vi "obstacle expansion.vi"() -> ()   [LabVIEW 2010]
uses:
  4-High Neurons/4.1.2-Act Neuron TD.ctl
  3.0 Flow Control/3.0 List of Loops.ctl
  3.0-Global.vi
panel:
  out "Input Act Neurons":T1
  out "Heartbeat":bool
  out "Dont Run!":bool
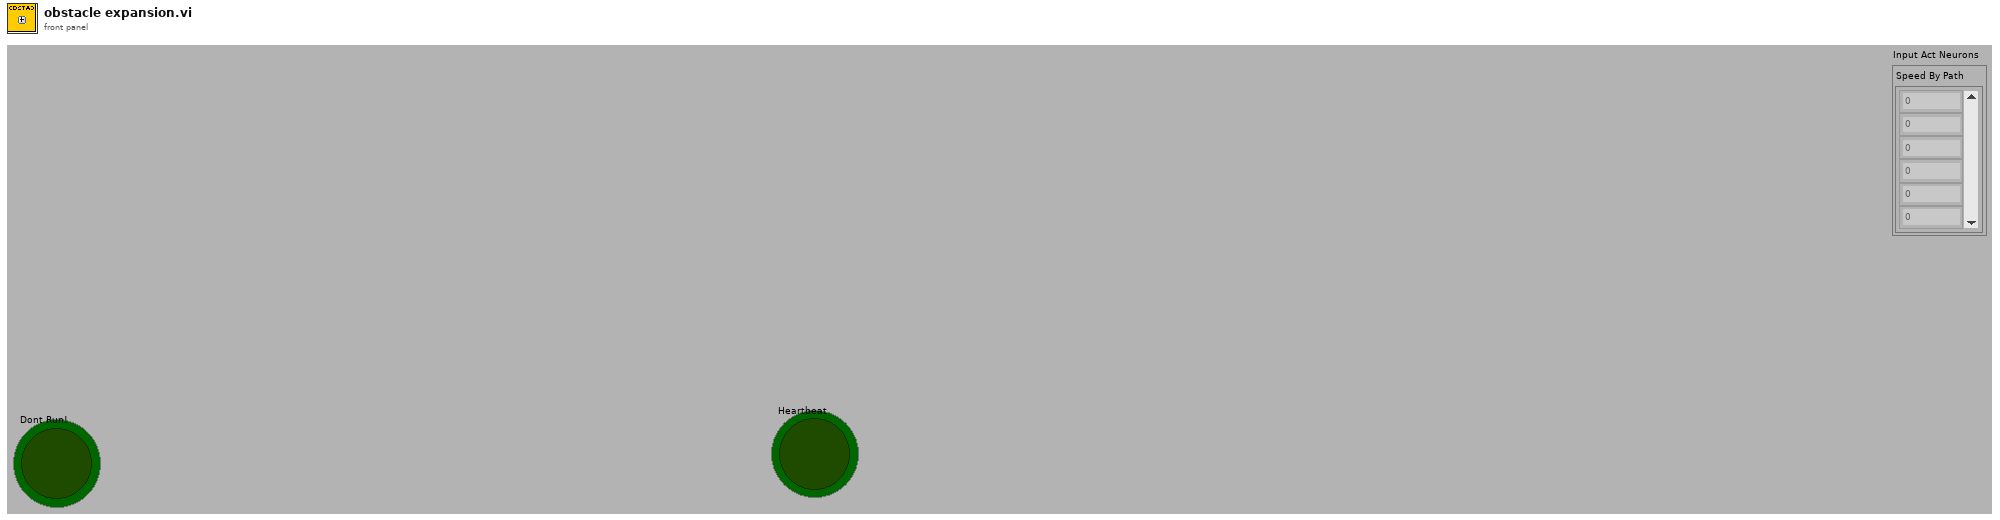
[diagram p1: front panel]
types:
  T1 = typedef "4.1.2-Act Neuron TD.ctl" = cluster{"Speed By Path":sgl[]}
  T2 = enum16{"Set Joystick", "Read Joystick", "Set Forebrain", "Read Forebrain", "Set Limbic", "Read Limbic", "Set Cerebellum", "Read Cerebellum", "Set Arbitrated", "Read Arbitrated", "Set LIDAR", "Read LIDAR"}
  T3 = typedef "3.0 List of Loops.ctl" = enum16{"3.0 State Update", "3.0 GUI", "3.1 Act", "3.1 4.7.1 Act UDP", "3.1 Joystick", "3.2 Where", "3.2 4.7.2 Where UDP", "3.3 What", "3.3 4.7.3 What UDP", "3.4 How", "3.4 4.7.4 How UDP", "3.5 Limbic", "3.8 TCP", "3.6 Cerebellum", "3.8 TCP Act"}
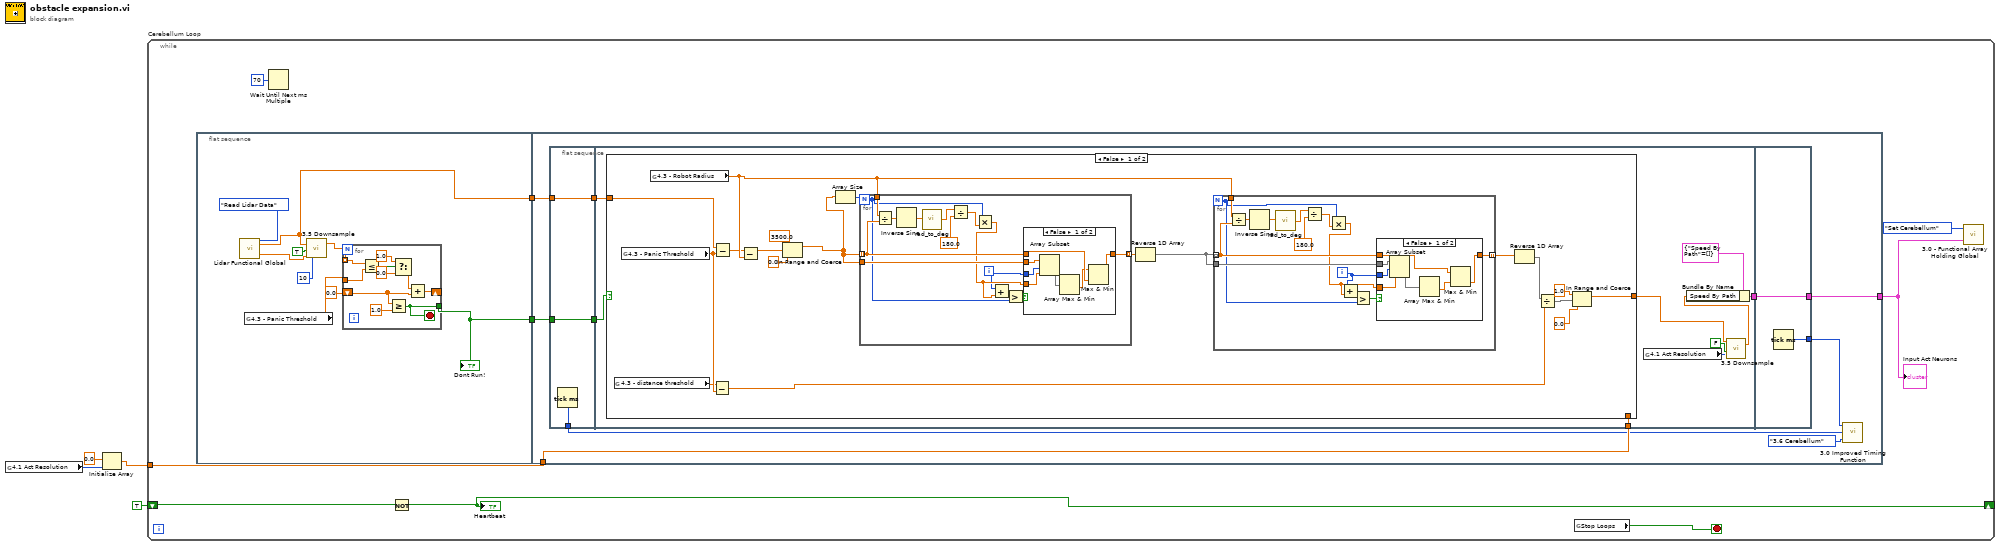
[diagram p0: block diagram]
diagram:
  n1 = global read "3.0-Global.vi" "4.1 Act Resolution"() -> (w2:u32)
  n2 = Initialize Array(0.0 ("element"), w2) -> (w1:dbl[])
  n3 = while "Cerebellum Loop" {
    shift-right: [w10] -> _
    shift-left: TRUE -> [w9]
    tunnel: w1 -> [w8]
    stop <- w11 stop-if-true
    n4 = flat-sequence {
      tunnel: [w15] -> w13
      tunnel: [w16] -> w12
      tunnel: w13 -> [w41]
      tunnel: w12 -> [w42]
      tunnel: w8 -> [w40]
      tunnel: [w39] -> w6
      frame #0 {
        n5 = call "Lidar Functional Global.vi"("Lidar Action"=enum16{"Set Lidar Data", "Read Lidar Data"}."Read Lidar Data") -> ("Lidar Angle Data Out (Degrees)"=w14:sgl[], "Lidar Magnitude Data Out (mm)"=w15:sgl[])  [unwired: 2 in]
        n6 = global read "3.0-Global.vi" "4.3 - Panic Threshold"() -> (w17:dbl)
        n7 = call "3.5 Downsample.vi"("Corresponding Input Array For Minimum"=w14, "Minimum?"=TRUE, "Numeric"=10, "Input Array"=w15) -> ("Output Array"=w19:sgl[])  [unwired: 1 out]
        n8 = for {
          shift-right: [w26] -> _
          shift-left: 0.0 -> [w25]
          tunnel: w19 -> [w32] mode=indexing
          tunnel: w17 -> [w31]
          tunnel: [w23] -> w16
          stop <- w23 stop-if-true
          n9 = Less Or Equal?(x=w32, y=w31) -> (x <= y?=w30:bool)
          n10 = Greater Or Equal?(x=w25, y=1.0) -> (x >= y?=w23:bool)
          n11 = Select(t=1.0, s=w30, f=0.0) -> (s? t:f=w27:dbl)
          n12 = Add(x=w27, y=w25) -> (x+y=w26:dbl)
        }
        "Dont Run!" <- w16
      }
      frame #1 {
        n13 = flat-sequence {
          tunnel: w41 -> [w44]
          tunnel: w42 -> [w45]
          tunnel: [w45] -> w37
          tunnel: [w44] -> w36
          tunnel: [w43] -> w33
          tunnel: w40 -> [w52]
          tunnel: [w50] -> w38
          tunnel: w37 -> [w54]
          tunnel: w36 -> [w53]
          tunnel: [w120] -> w39
          tunnel: w38 -> [w120]
          tunnel: [w119] -> w34
          frame #0 {
            n14 = Tick Count (ms)() -> (millisecond timer value=w43:u32)
          }
          frame #1 {
            n15 = case shown="False" w54 {
              tunnel: w53 -> [w71 _]
              tunnel: [w55 w118] -> w47
              tunnel: w52 -> [_ w118]
              frame False {
                n16 = global read "3.0-Global.vi" "4.3 - distance threshold"() -> (w72:dbl)
                n17 = global read "3.0-Global.vi" "4.3 - Panic Threshold"() -> (w73:dbl)
                n18 = global read "3.0-Global.vi" "4.3 - Robot Radius"() -> (w63:dbl)
                n19 = Subtract(x=w72, y=w73) -> (x-y=w61:dbl)
                n20 = Subtract(x=w71, y=w73) -> (x-y=w62:dbl[])
                n21 = Subtract(x=w62, y=w63) -> (x-y=w59:dbl[])
                n22 = In Range and Coerce(upper limit=3500.0, x=w59, lower limit=0.0) -> (coerced(x)=w56:dbl[])  [unwired: 1 out]
                n23 = Array Size(array=w56) -> (size(s)=w70:i32)
                n24 = for {
                  N: w70 -> [w96]
                  tunnel: w56 -> [w106] mode=indexing
                  tunnel: w56 -> [w109]
                  tunnel: [w100] -> w60 mode=indexing
                  tunnel: w63 -> [w107]
                  i -> [w98]
                  n25 = Divide(x=w107, y=w106) -> (x/y=w108:dbl)
                  n26 = Inverse Sine(1:w108) -> (0:w104:dbl)
                  n27 = call "rad_to_deg.vi"("Radians"=w104) -> ("Degrees"=w102:dbl)
                  n28 = Divide(x=w102, y=180.0 ("x")) -> (x/y=w103:dbl)
                  n29 = Multiply(x=w96, y=w103) -> (x*y=w99:dbl)
                  n30 = Add(x=w98, y=w99) -> (x+y=w97:dbl)
                  n31 = Greater?(x=w97, y=w96) -> (0:w101:bool)
                  n32 = case shown="False" w101 {
                    tunnel: w106 -> [w116 w117]
                    tunnel: [w113 w117] -> w100
                    tunnel: w98 -> [w115 _]
                    tunnel: w109 -> [w114 _]
                    tunnel: w99 -> [w112 _]
                    frame False {
                      n33 = Array Subset(array=w114, index=w115, length=w112) -> (w110:dbl[])
                      n34 = Array Max & Min(array=w110) -> (min value=w111:dbl)  [unwired: 3 out]
                      n35 = Max & Min(x=w111, y=w116) -> (min(x,y)=w113:dbl)  [unwired: 1 out]
                    }
                    frame True {
                    }
                  }
                }
                n36 = Reverse 1D Array(array=w60) -> (reversed array=w67:dbl[])
                n37 = for {
                  N -> [w74]
                  tunnel: w67 -> [w83] mode=indexing
                  tunnel: w67 -> [w86]
                  tunnel: [w87] -> w64 mode=indexing
                  tunnel: w63 -> [w84]
                  i -> [w77]
                  n38 = Divide(x=w84, y=w83) -> (x/y=w85:dbl)
                  n39 = Inverse Sine(1:w85) -> (0:w81:dbl)
                  n40 = call "rad_to_deg.vi"("Radians"=w81) -> ("Degrees"=w79:dbl)
                  n41 = Divide(x=w79, y=180.0 ("x")) -> (x/y=w80:dbl)
                  n42 = Multiply(x=w74, y=w80) -> (x*y=w76:dbl)
                  n43 = Add(x=w77, y=w76) -> (x+y=w75:dbl)
                  n44 = Greater?(x=w75, y=w74) -> (0:w78:bool)
                  n45 = case shown="False" w78 {
                    tunnel: w83 -> [w90 w95]
                    tunnel: [w92 w95] -> w87
                    tunnel: w77 -> [w94 _]
                    tunnel: w86 -> [w93 _]
                    tunnel: w76 -> [w91 _]
                    frame False {
                      n46 = Array Subset(array=w93, index=w94, length=w91) -> (w89:dbl[])
                      n47 = Array Max & Min(array=w89) -> (min value=w88:dbl)  [unwired: 3 out]
                      n48 = Max & Min(x=w90, y=w88) -> (min(x,y)=w92:dbl)  [unwired: 1 out]
                    }
                    frame True {
                    }
                  }
                }
                n49 = Reverse 1D Array(array=w64) -> (reversed array=w66:dbl[])
                n50 = Divide(x=w66, y=w61) -> (x/y=w65:dbl[])
                n51 = In Range and Coerce(upper limit=1.0, x=w65, lower limit=0.0) -> (coerced(x)=w55:dbl[])  [unwired: 1 out]
              }
              frame True {
              }
            }
            n52 = global read "3.0-Global.vi" "4.1 Act Resolution"() -> (w48:u32)
            n53 = call "3.5 Downsample.vi"("Minimum?"=FALSE, "Numeric"=w48, "Input Array"=w47) -> ("Output Array"=w46:sgl[])  [unwired: 1 in, 1 out]
            n54 = Bundle By Name(cluster=T1 {"Speed By Path"=[]} ("Input Act Neurons"), "Speed By Path"=w46) -> (w50:T1)
          }
          frame #2 {
            n55 = Tick Count (ms)() -> (millisecond timer value=w119:u32)
          }
        }
        n56 = call "3.0 Improved Timing Function.vi"("Loop"=3.0_List_of_Loops."3.6 Cerebellum", "Start"=w33, "End"=w34) -> ()  [unwired: 1 in]
      }
    }
    n57 = Wait Until Next ms Multiple(millisecond multiple=u32 70) -> ()  [unwired: 1 out]
    n58 = Not(x=w9) -> (.not. x?=w10:bool)
    "Heartbeat" <- w10
    n59 = global read "3.0-Global.vi" "Stop Loops"() -> (w11:bool)
    n60 = call "3.0 - Functional Array Holding Global.vi"("Input Act Neurons"=w6, "Mode"=T2."Set Cerebellum") -> ()  [unwired: 1 out]
    "Input Act Neurons" <- w6
  }
